vi "Thermometer.vi"(11 "Temp Scale":bool) -> (3 "Temperature":dbl(slide) scale=0.0..100.0)   [LabVIEW 2019]
doc: "This VI measures temperature using the temp.vi as input"
panel:
  # "deg C"
  # "deg F"
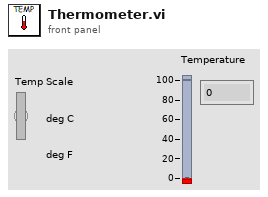
[diagram p1: front panel]
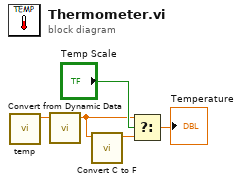
[diagram p0: block diagram]
diagram:
  n1 = call "temp.vi"() -> ("voltage"=w2:dbl)  [unwired: 6 in, 1 out]
  n2 = call "Convert from Dynamic Data"("Dynamic Data Type"=w2) -> ("Scalar"=w1:dbl)  [unwired: 3 in]
  n3 = call "Convert C to F.vi"("Celcius"=w1) -> ("Farenheit"=w3:dbl)  [unwired: 10 in]
  n4 = Select(t=w1, s="Temp Scale", f=w3) -> (s? t:f=→"Temperature":dbl)
